vi "automatico.vi"() -> ()   [LabVIEW 2011]
uses:
  <vilib>/Analysis/Matrix/Numeric/Conversions/Array To Matrix - RA.vi
  <vilib>/Analysis/Matrix/Numeric/Conversions/Matrix To Array - RM.vi
  <vilib>/Analysis/Matrix/NI_Matrix.lvlib
  <vilib>/Analysis/NI_AALBase.lvlib
  <vilib>/Analysis/NI_AALPro.lvlib
panel:
  in  "Numeric 2":i32
  in  "Play Button":bool
  out "time stamp":timestamp format="%<%.3X>T"
  in  "Numeric":i32=5
  out "Time cinetica":dbl format="%0.2f"
  in  "time subarray":dbl[](array[numeric])
  out "Elapsed Time (sec)":dbl format="%.1f"
  in  "T subarray 2":dbl[](array[numeric])
  in  "P T  index":i32
  in  "P subarray":dbl[](array[numeric])
  out "Vol Ref":dbl(slide) scale=0.0..50.0 scale format="%#_4f"
  out "P cinetica mean":dbl format="%0.2f"
  out "T cinetica mean 2":dbl format="%0.2f"
  in  "clear":bool
  out "Automatico":dynamicdata(graph)
  out "Linear P":T1(graph)
  out "Linear T":T1(graph)
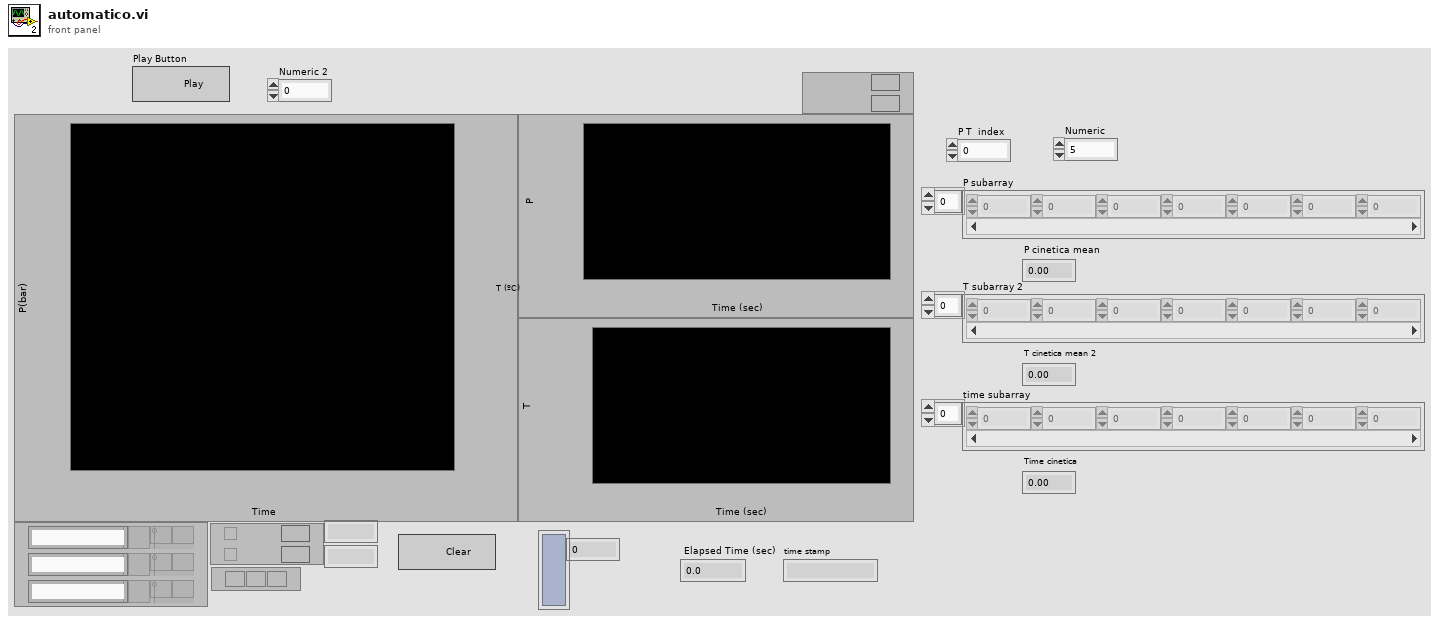
[diagram p1: front panel]
types:
  T1 = cluster{"Real 2D Array":dbl[], "Best Linear Fit":dbl[]}[]
  T2 = typedef "NI_Matrix.lvlib/RealMatrix.ctl" = dbl[][]
  T3 = cluster{"Real 2D Array":dbl[], "Real 2D Array":dbl[]}
  T4 = cluster{"Real 2D Array":dbl[], "Best Linear Fit":dbl[]}
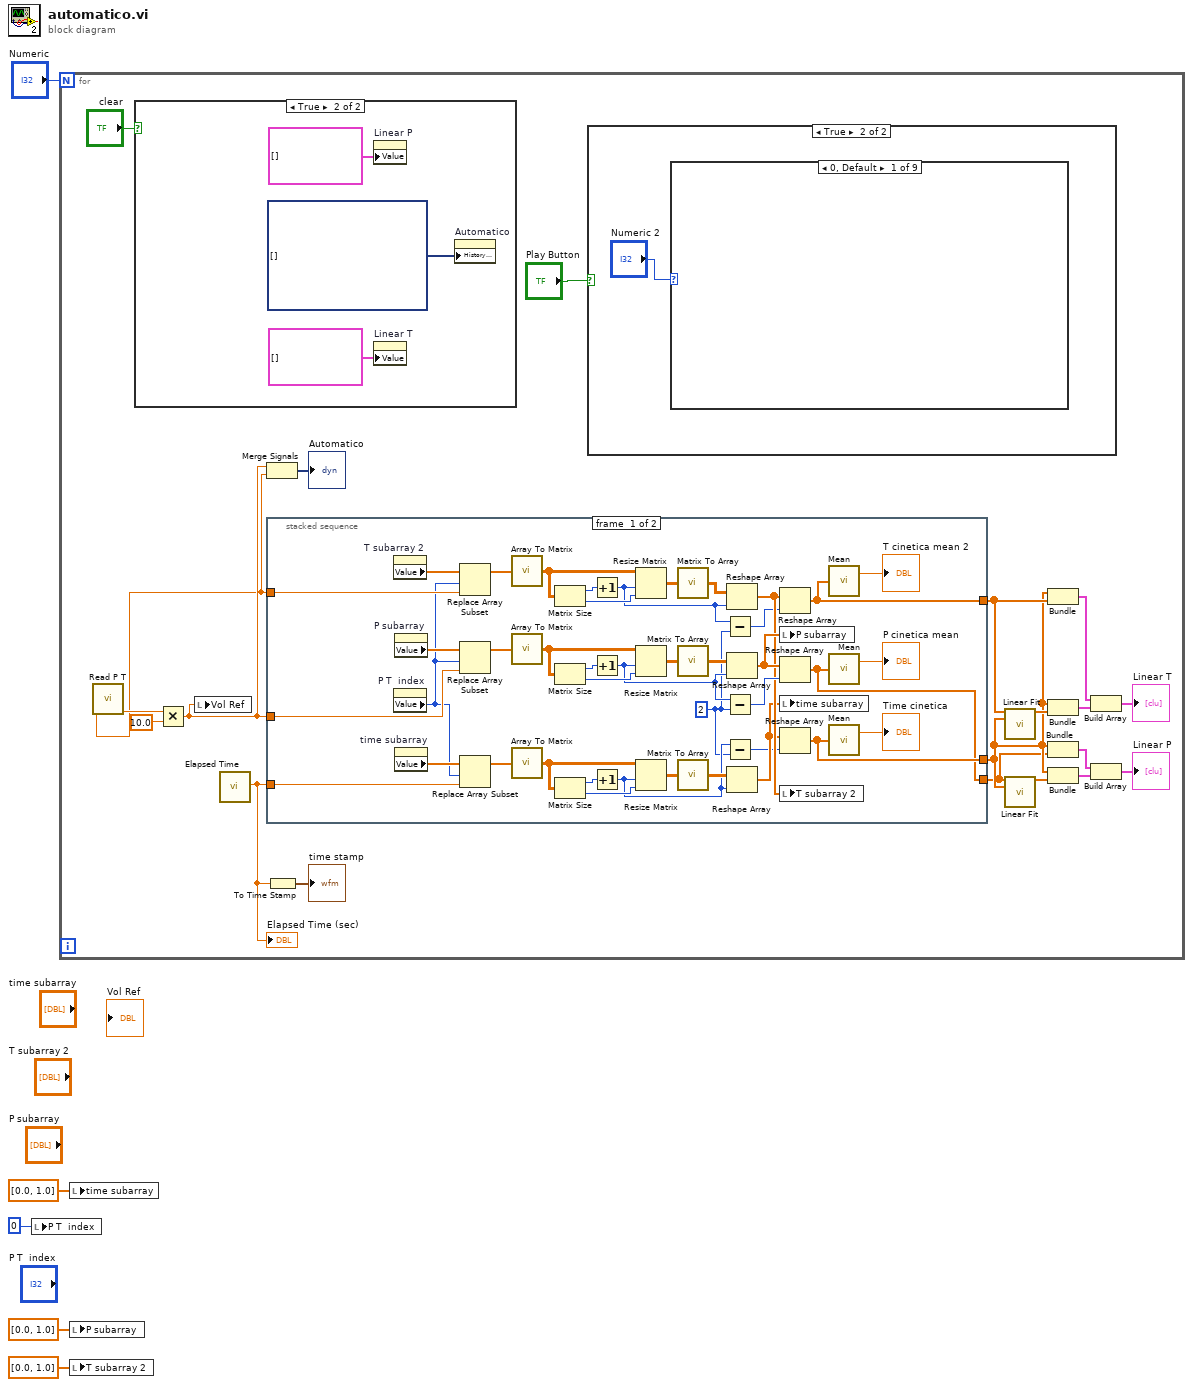
[diagram p0: block diagram]
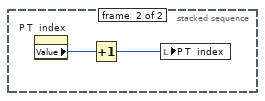
[diagram p11: hidden frame]
diagram:
  n1 = local write "P T  index"(0 ("P T  index")) -> ()
  n2 = for {
    N: "Numeric" -> [_]
    n3 = call "Read P T.vi"() -> ("P Set 2 Output 2"=w23:dbl, "T Set 2 Output"=w21:dbl)  [unwired: 4 in, 6 out]
    n4 = case shown="True" "clear" {
      frame False {
      }
      frame True {
        n5 = property on="Linear P" class="XYGraph (strict)"("Value"=T1 [] ("Linear P")) -> ()  [unwired: 2 in, 2 out]
        n6 = property on="Linear T" class="XYGraph (strict)"("Value"=T1 [] ("Linear T")) -> ()  [unwired: 2 in, 2 out]
        n7 = property on="Automatico" class="WFChart (strict)"("History Data"=dynamicdata[] []) -> ()  [unwired: 2 in, 2 out]
      }
    }
    n8 = Multiply(x=w23, y=10.0) -> (x*y=w22:dbl)
    n9 = local write "Vol Ref"(w22) -> ()
    n10 = call "Elapsed Time"() -> ("Elapsed Time (s)"=w8:dbl)  [unwired: 12 in, 7 out]
    "Elapsed Time (sec)" <- w8
    n11 = Merge Signals(w22, w21) -> (→"Automatico":dynamicdata)
    n12 = stacked-sequence {
      tunnel: w22 -> [w62 _]
      tunnel: w21 -> [w46 _]
      tunnel: [w27 _] -> w10
      tunnel: [w43 _] -> w17
      tunnel: w8 -> [w30 _]
      tunnel: [w28 _] -> w11
      frame #0 {
        w29 = 2 ("y")
        n13 = property on="T subarray 2" class="Arr (strict)"() -> ("Value"=w53:dbl[])  [unwired: 2 in, 2 out]
        n14 = property on="P T  index" class="DigNum (strict)"() -> ("Value"=w31:i32)  [unwired: 2 in, 2 out]
        n15 = property on="P subarray" class="Arr (strict)"() -> ("Value"=w64:dbl[])  [unwired: 2 in, 2 out]
        n16 = property on="time subarray" class="Arr (strict)"() -> ("Value"=w39:dbl[])  [unwired: 2 in, 2 out]
        n17 = Replace Array Subset(array=w53, new element=w46, index=w31) -> (w44:dbl[])
        n18 = Replace Array Subset(array=w64, new element=w62, index=w31) -> (w45:dbl[])
        n19 = Replace Array Subset(array=w39, new element=w30, index=w31) -> (w32:dbl[])
        n20 = call-poly <vilib>:"Array To Matrix.vi"("Real 1D Array"=w44) -> ("Real Matrix (Column Vector)"=w56:T2)
        n21 = call-poly <vilib>:"Array To Matrix.vi"("Real 1D Array"=w45) -> ("Real Matrix (Column Vector)"=w67:T2)
        n22 = call-poly <vilib>:"Array To Matrix.vi"("Real 1D Array"=w32) -> ("Real Matrix (Column Vector)"=w42:T2)
        n23 = Matrix Size(0:w56) -> (1:w55:i32, 2:w54:i32)
        n24 = Matrix Size(0:w67) -> (1:w66:i32, 2:w65:i32)
        n25 = Matrix Size(0:w42) -> (1:w41:i32, 2:w40:i32)
        n26 = Increment(x=w55) -> (x+1=w47:i32)
        n27 = Increment(x=w66) -> (x+1=w57:i32)
        n28 = Increment(x=w41) -> (x+1=w33:i32)
        n29 = Resize Matrix(1:w54, 2:w47, 4:w56) -> (0:w52:T2)
        n30 = Resize Matrix(1:w65, 2:w57, 4:w67) -> (0:w63:T2)
        n31 = Resize Matrix(1:w40, 2:w33, 4:w42) -> (0:w38:T2)
        n32 = call-poly <vilib>:"Matrix To Array.vi"("Real Matrix"=w52) -> ("Real 2D Array"=w50:dbl[][])
        n33 = call-poly <vilib>:"Matrix To Array.vi"("Real Matrix"=w63) -> ("Real 2D Array"=w60:dbl[][])
        n34 = call-poly <vilib>:"Matrix To Array.vi"("Real Matrix"=w38) -> ("Real 2D Array"=w36:dbl[][])
        n35 = Subtract(x=w47, y=w29) -> (x-y=w48:i32)
        n36 = Subtract(x=w57, y=w29) -> (x-y=w58:i32)
        n37 = Subtract(x=w33, y=w29) -> (x-y=w34:i32)
        n38 = Reshape Array(w50, w47) -> (w49:dbl[])
        n39 = Reshape Array(w60, w57) -> (w59:dbl[])
        n40 = Reshape Array(w36, w33) -> (w35:dbl[])
        n41 = Reshape Array(w49, w48) -> (w43:dbl[])
        n42 = local write "P subarray"(w59) -> ()
        n43 = Reshape Array(w59, w58) -> (w27:dbl[])
        n44 = local write "time subarray"(w35) -> ()
        n45 = Reshape Array(w35, w34) -> (w28:dbl[])
        n46 = local write "T subarray 2"(w49) -> ()
        n47 = call <vilib>:"Mean.vi"("X"=w43) -> ("mean"=→"T cinetica mean 2":dbl)  [unwired: 1 out]
        n48 = call <vilib>:"Mean.vi"("X"=w27) -> ("mean"=→"P cinetica mean":dbl)  [unwired: 1 out]
        n49 = call <vilib>:"Mean.vi"("X"=w28) -> ("mean"=→"Time cinetica":dbl)  [unwired: 1 out]
      }
      frame #1 {
        n50 = property on="P T  index" class="DigNum (strict)"() -> ("Value"=w69:i32)  [unwired: 2 in, 2 out]
        n51 = Increment(x=w69) -> (x+1=w68:i32)
        n52 = local write "P T  index"(w68) -> ()
      }
    }
    n53 = To Time Stamp(1:w8) -> (0:→"time stamp":timestamp)
    n54 = case shown="True" "Play Button" {
      frame False {
      }
      frame True {
        n55 = case shown="0, Default" "Numeric 2" {
          frame 0, Default {
          }
          frame 1 {
          }
          frame 2 {
          }
          frame 3 {
          }
          frame 4 {
          }
          frame 5 {
          }
          frame 6 {
          }
          frame 7 {
          }
          frame 8 {
          }
        }
      }
    }
    n56 = call <vilib>:"Linear Fit.vi"("Y"=w17, "X"=w11) -> ("Best Linear Fit"=w16:dbl[])  [unwired: 9 in, 4 out]
    n57 = call <vilib>:"Linear Fit.vi"("Y"=w10, "X"=w11) -> ("Best Linear Fit"=w9:dbl[])  [unwired: 9 in, 4 out]
    n58 = Bundle("Real 2D Array"=w11, "Real 2D Array"=w17) -> (w14:T3)  [unwired: 1 in]
    n59 = Bundle("Real 2D Array"=w11, "Best Linear Fit"=w16) -> (w15:T4)  [unwired: 1 in]
    n60 = Bundle("Real 2D Array"=w11, "Real 2D Array"=w10) -> (w13:T3)  [unwired: 1 in]
    n61 = Bundle("Real 2D Array"=w11, "Best Linear Fit"=w9) -> (w12:T4)  [unwired: 1 in]
    n62 = Build Array(w14, w15) -> (→"Linear T":T1)
    n63 = Build Array(w13, w12) -> (→"Linear P":T1)
  }
  n64 = local write "time subarray"(dbl[] [0.0, 1.0] ("subarray")) -> ()
  n65 = local write "P subarray"(dbl[] [0.0, 1.0] ("subarray")) -> ()
  n66 = local write "T subarray 2"(dbl[] [0.0, 1.0] ("subarray")) -> ()
